vi "intMaxMin.vi"(8 "Error in (no error)":errorcluster, 10 "Int2 in":refnum<class "IntClass.lvclass">, 11 "Int1 in":refnum<class "IntClass.lvclass">) -> (0 "Error out":errorcluster, 1 "Timing":u32, 2 "Min":refnum<class "IntClass.lvclass">, 3 "Max":refnum<class "IntClass.lvclass">)   [LabVIEW 2011, in "IntClass.lvclass"]
uses:
  IntClass.lvclass
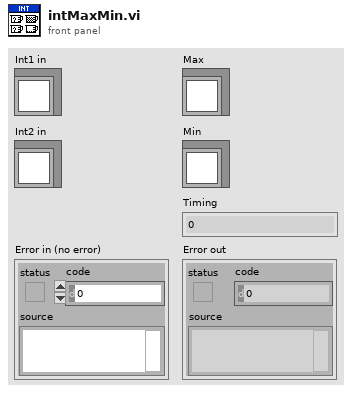
[diagram p1: front panel]
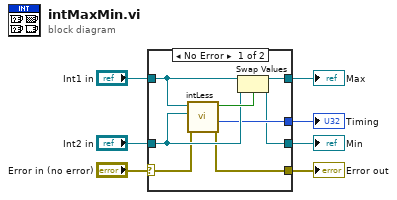
[diagram p0: block diagram]
diagram:
  n1 = case shown="No Error" "Error in (no error)" {
    selector: "Error in (no error)" -> [w11 w16]
    tunnel: "Int1 in" -> [w14 _]
    tunnel: "Int2 in" -> [w13 _]
    tunnel: [w12 w16] -> w4
    tunnel: [w10 _] -> w3
    tunnel: [w9 _] -> w2
    tunnel: [w8 _] -> w1
    frame No Error {
      n2 = call "intLess.vi"("Error in (no error)"=w11, "Int2 in"=w13, "Int1 in"=w14) -> ("Error out"=w12:errorcluster, "Timing"=w10:u32, "Int1 < Int2?"=w15:bool)  [unwired: 6 in]
      n3 = Swap Values(12:w14, 13:w15, 14:w13) -> (1:w9:refnum<class "IntClass.lvclass">, 3:w8:refnum<class "IntClass.lvclass">)
    }
    frame Error {
    }
  }
  "Error out" <- w4
  "Timing" <- w3
  "Max" <- w2
  "Min" <- w1
